vi "resistanceCheck_RS485.vi"() -> ()   [LabVIEW 2018]
panel:
  in  "stop":bool
  out "ADC value":dbl
  out "resistance485Array":dbl[](array[numeric])
  out "overCurrent":bool
  out "QuickResistance":bool=TRUE
  in  "stopR":bool
  out "RESISTANCE/CURRENT":cluster{dbl, dbl}(graph)
  out "Ipeak":string
  out "IRun":string
  out "Value":dbl
  out "Press Next":dbl
  out "cycle":dbl
  out "No Keys":bool
  out "steps/button Array":dbl[][](array[numeric])
  in  "VISA Refnum in":refnum<visa-resource-name>
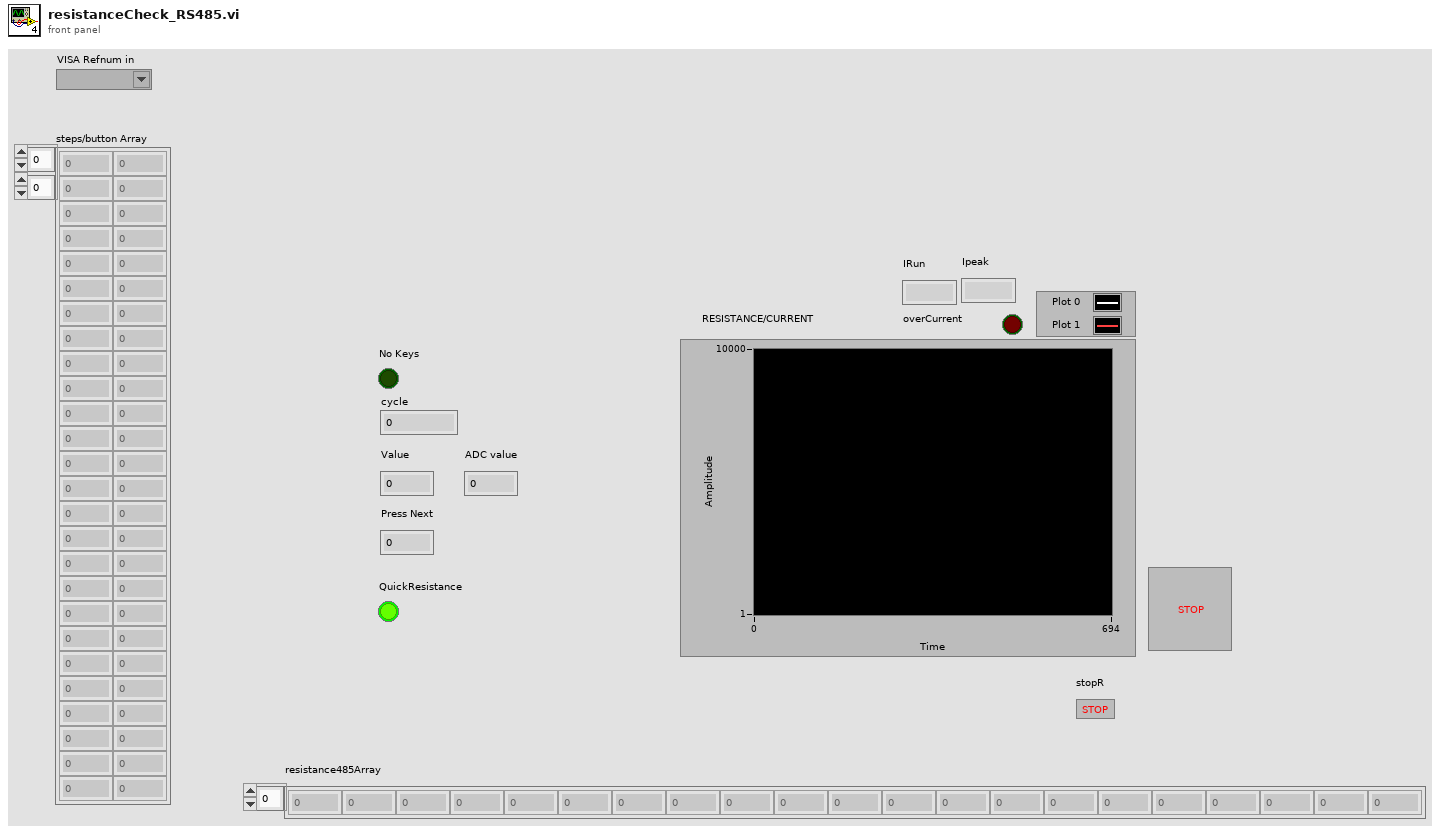
[diagram p1: front panel]
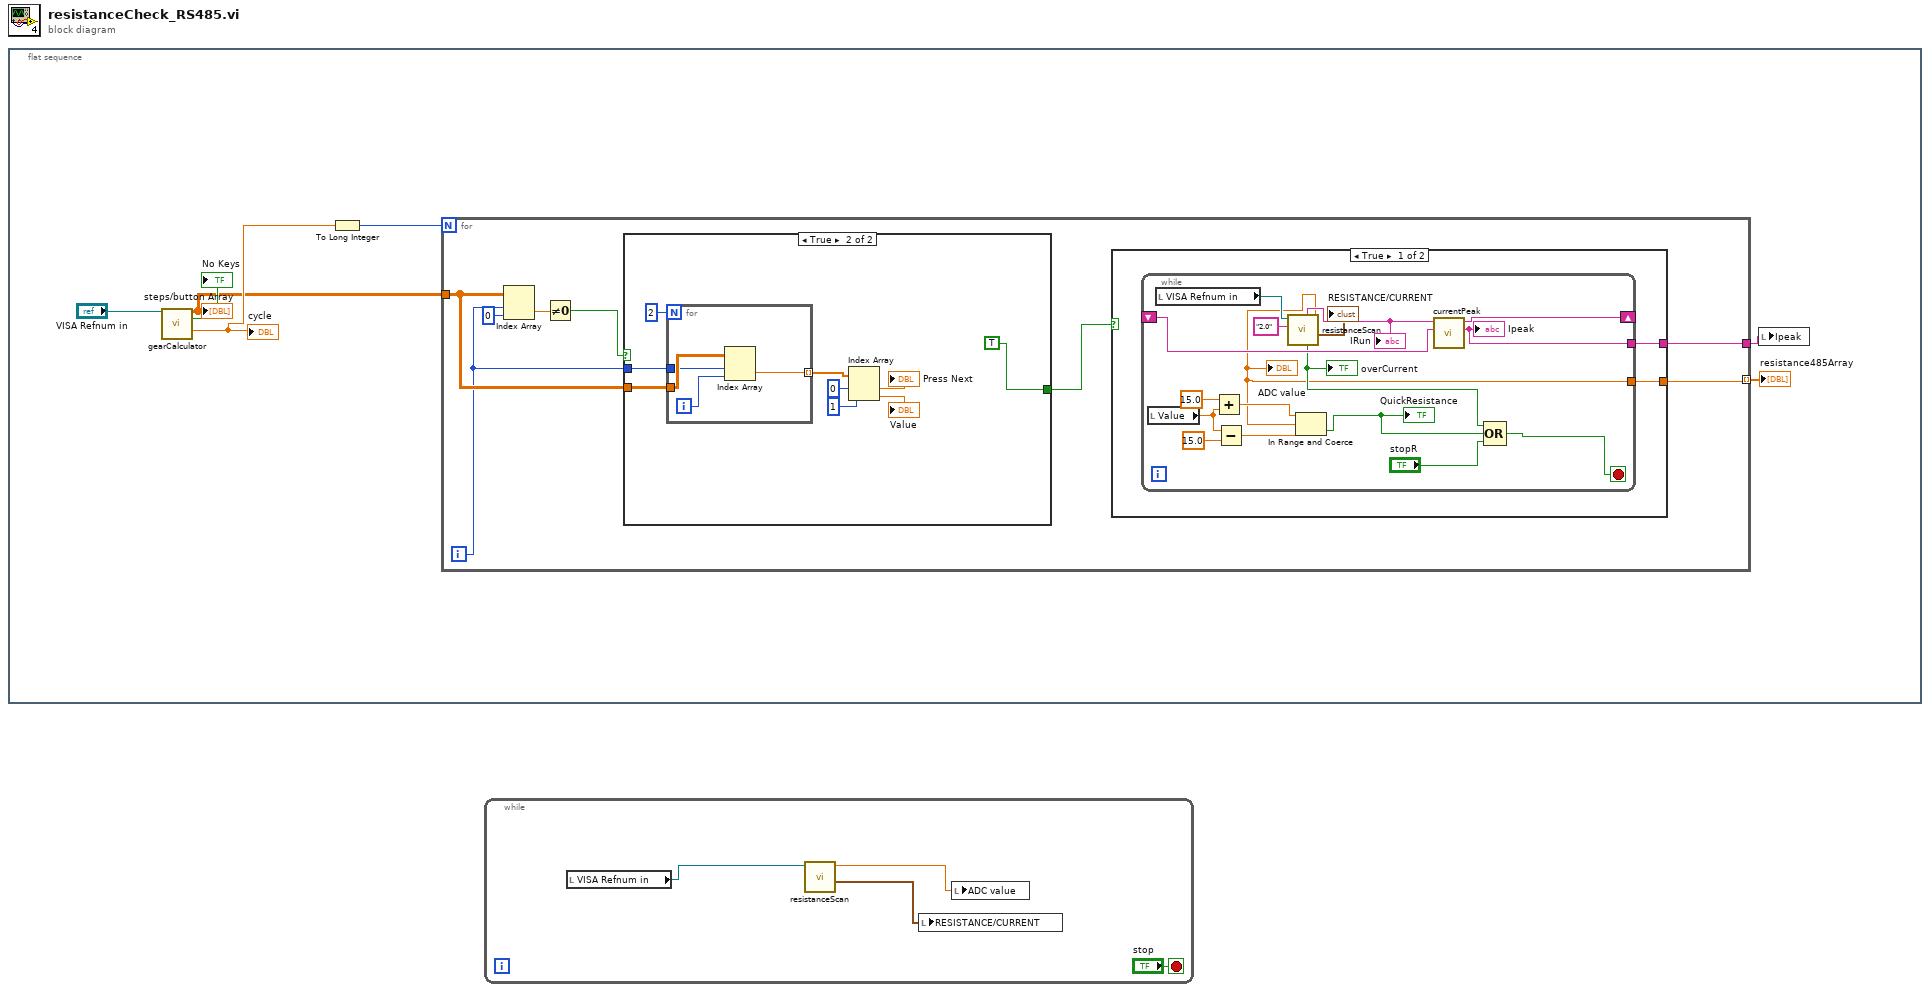
[diagram p0: block diagram]
diagram:
  n1 = flat-sequence {
    frame #0 {
      n2 = call "gearCalculator.vi"("VISA Refnum in"="VISA Refnum in") -> ("steps/button Array"=w3:dbl[][], "No Keys"=→"No Keys":bool, "cycle"=w5:dbl)  [unwired: 10 in, 2 out]
      "steps/button Array" <- w3
      "cycle" <- w5
      n3 = To Long Integer(number=w5) -> (32bit integer=w4:i32)
      n4 = for {
        N: w4 -> [_]
        tunnel: w3 -> [w12]
        tunnel: [w9] -> w2 mode=indexing
        tunnel: [w8] -> w1
        i -> [w11]
        n5 = Index Array(array=w12, index (row)=w11, index (col)=0 ("disabled index (col)")) -> (element=w15:dbl)
        n6 = Not Equal To 0?(x=w15) -> (x != 0?=w14:bool)
        n7 = case shown="True" w14 {
          selector: w14 -> [w35 _]
          tunnel: w12 -> [_ w43]
          tunnel: w11 -> [_ w42]
          tunnel: [w35 TRUE] -> w10
          frame False {
          }
          frame True {
            n8 = for {
              N: 2 -> [_]
              tunnel: w43 -> [w48]
              tunnel: w42 -> [w46]
              tunnel: [w45] -> w41 mode=indexing
              i -> [w47]
              n9 = Index Array(array=w48, index (row)=w46, index (col)=w47) -> (element=w45:dbl)
            }
            n10 = Index Array(array=w41, index #1=0 ("index"), index #2=1 ("index")) -> (element #1=→"Press Next":dbl, element #2=→"Value":dbl)
          }
        }
        n11 = case shown="True" w10 {
          tunnel: [w17 _] -> w9
          tunnel: [w16 _] -> w8
          frame True {
            n12 = while {
              shift-right: [w31] -> _
              shift-left: _ -> [w30]
              tunnel: [w19] -> w17
              tunnel: [w18] -> w16
              stop <- w28 stop-if-true
              n13 = local read "Value"() -> (w24:dbl)
              n14 = local read "VISA Refnum in"() -> (w33:refnum<visa-resource-name>)
              n15 = Add(x=15.0, y=w24) -> (x+y=w20:dbl)
              n16 = Subtract(x=w24, y=15.0) -> (x-y=w21:dbl)
              n17 = call "resistanceScan.vi"("Imax"="2.0", "VISA Refnum in"=w33) -> ("RESISTANCE/CURRENT"=→"RESISTANCE/CURRENT":cluster{dbl, dbl}, "ADC value"=w19:dbl, "overCurrent"=w25:bool, "Istring#"=w32:string)  [unwired: 5 in, 1 out]
              "IRun" <- w32
              "overCurrent" <- w25
              "ADC value" <- w19
              n18 = In Range and Coerce(upper limit=w20, x=w19, lower limit=w21) -> (In Range?=w26:bool)  [unwired: 1 out]
              "QuickResistance" <- w26
              n19 = call "currentPeak.vi"("Istring# change"=w30, "Istring# scan"=w32) -> ("Ipeak"=w18:string, "Irun"=w31:string)  [unwired: 7 in, 1 out]
              "Ipeak" <- w18
              n20 = Compound Arithmetic op=OR(w25, w26, "stopR") -> (w28:bool)
            }
          }
          frame False {
          }
        }
      }
      "resistance485Array" <- w2
      n21 = local write "Ipeak"(w1) -> ()
    }
  }
  n22 = while {
    stop <- "stop" stop-if-true
    n23 = local read "VISA Refnum in"() -> (w49:refnum<visa-resource-name>)
    n24 = call "resistanceScan.vi"("VISA Refnum in"=w49) -> ("RESISTANCE/CURRENT"=w52:cluster{dbl, dbl}, "ADC value"=w51:dbl)  [unwired: 6 in, 3 out]
    n25 = local write "RESISTANCE/CURRENT"(w52) -> ()
    n26 = local write "ADC value"(w51) -> ()
  }
